vi "Picture_Init_Size.vi"(8 "Input Cluster":T6) -> (0 "Output Cluster":T6, 3 "Boolean":bool)   [LabVIEW 2009]
uses:
  atmcd32d.llb/AcquisitionMode_mode typedef.ctl
  atmcd32d.llb/ReadMode_mode typedef.ctl
  atmcd32d.llb/TriggerMode_mode typedef.ctl
  atmcd32d.llb/Shutter_type typedef.ctl
  atmcd32d.llb/Shutter_mode typedef.ctl
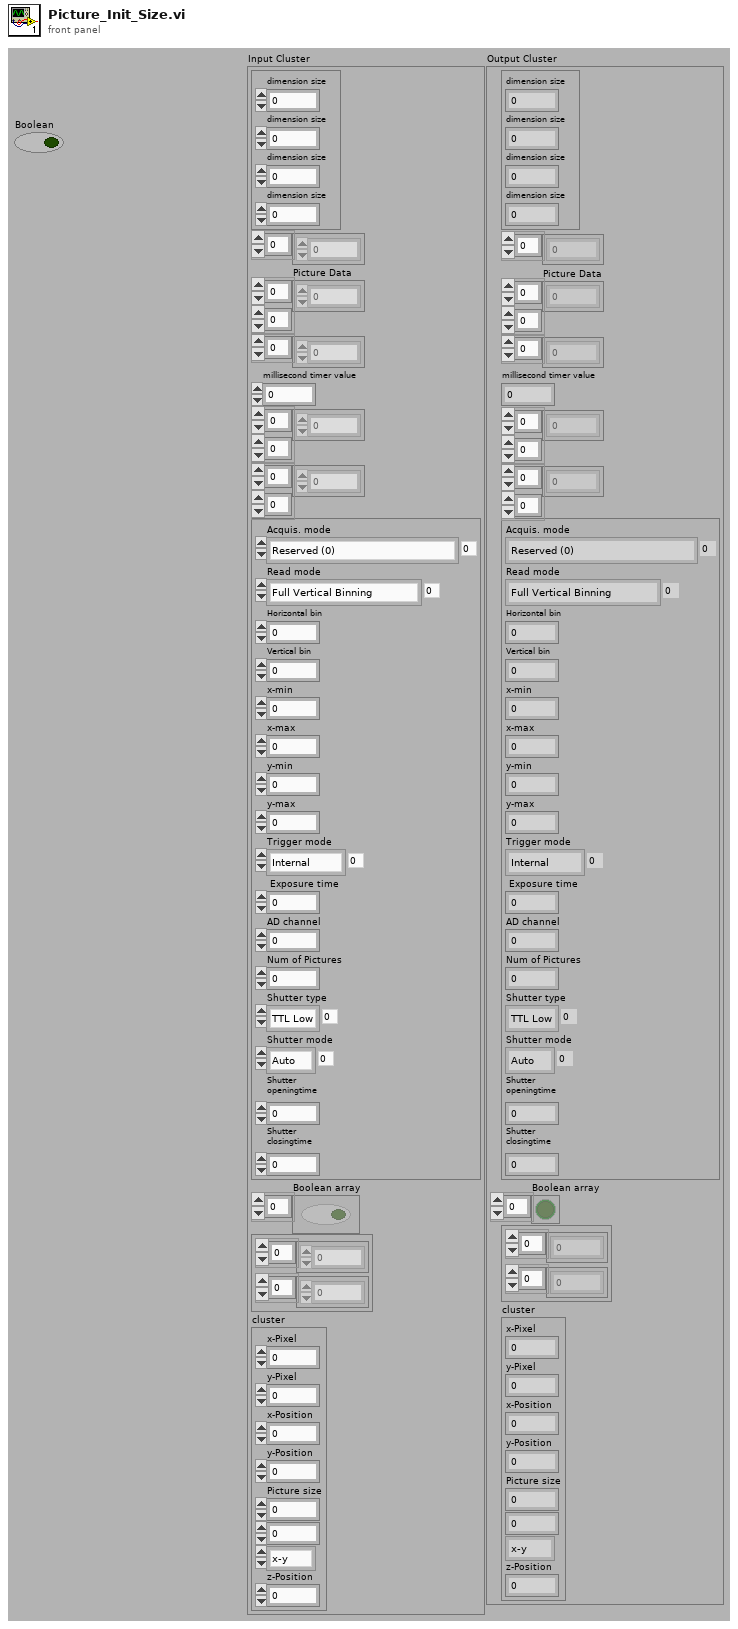
[diagram p1: front panel]
types:
  T1 = typedef "AcquisitionMode_mode typedef.ctl" = enum16{"Reserved (0)", "Single Scan", "Accumulate", "Kinetics", "Fast Kinetics", "Run Till Abort", "Reserved (6)", "Reserved (7)", "Reserved (8)", "Time Delayed Integration"}
  T2 = typedef "ReadMode_mode typedef.ctl" = enum16{"Full Vertical Binning", "Multi-Track", "Random-Track", "Single-Track", "Image"}
  T3 = typedef "TriggerMode_mode typedef.ctl" = enum16{"Internal", "External", "N/A (2)", "N/A (3)", "N/A (4)", "N/A (5)", "External Start"}
  T4 = typedef "Shutter_type typedef.ctl" = enum16{"TTL Low", "TTL High"}
  T5 = typedef "Shutter_mode typedef.ctl" = enum16{"Auto", "Open", "Close"}
  T6 = cluster{cluster{"dimension size":i32, "dimension size":i32, "dimension size":i32, "dimension size":i32}, i32[], "Picture Data":dbl[][], u32[], "millisecond timer value":u32, dbl[][], i32[][], cluster{"Acquis. mode":T1, "Read mode":T2, "Horizontal bin":i32, "Vertical bin":i32, "x-min":i32, "x-max":i32, "y-min":i32, "y-max":i32, "Trigger mode":T3, " Exposure time":sgl, "AD channel":i32, "Num of Pictures":i32, "Shutter type":T4, "Shutter mode":T5, "Shutter\nopeningtime":i32, "Shutter\nclosingtime":i32}, "Boolean array":bool[], cluster{dbl[], dbl[]}, "cluster":cluster{"x-Pixel":u16, "y-Pixel":u16, "x-Position":dbl, "y-Position":dbl, "Picture size":dbl, dbl, enum32{"x-y", "x-z", "y-z"}, "z-Position":dbl}}
  T7 = cluster{"x-Pixel":u16, "y-Pixel":u16, "x-Position":dbl, "y-Position":dbl, "Picture size":dbl, dbl, enum32{"x-y", "x-z", "y-z"}, "z-Position":dbl}
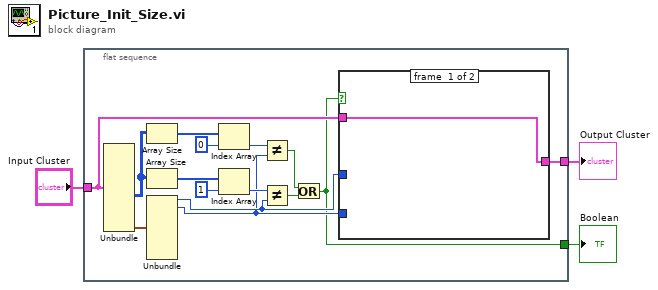
[diagram p0: block diagram]
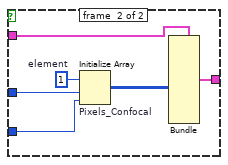
[diagram p2: hidden frame]
diagram:
  n1 = flat-sequence {
    tunnel: "Input Cluster" -> [w7]
    tunnel: [w6] -> w2
    tunnel: [w5] -> w3
    frame #0 {
      n2 = Unbundle(w7) -> (w13:i32[][], "cluster"=w4:T7)  [unwired: 9 out]
      n3 = Array Size(array=w13) -> (size(s)=w15:i32[])
      n4 = Array Size(array=w13) -> (size(s)=w18:i32[])
      n5 = Unbundle(w4) -> ("x-Pixel"=w9:u16, "y-Pixel"=w8:u16)  [unwired: 6 out]
      n6 = Index Array(array=w15, index=0) -> (element=w12:i32)
      n7 = Index Array(array=w18, index=1) -> (element=w16:i32)
      n8 = Not Equal?(x=w12, y=w8) -> (x != y?=w11:bool)
      n9 = Not Equal?(x=w16, y=w9) -> (x != y?=w10:bool)
      n10 = Or(x=w11, y=w10) -> (x .or. y?=w5:bool)
      n11 = case shown="True" w5 {
        tunnel: w9 -> [_ w24]
        tunnel: w8 -> [_ w23]
        tunnel: w7 -> [w19 w22]
        tunnel: [w19 w20] -> w6
        frame #0 {
        }
        frame #1 {
          w25 = 1  # element
          n12 = Initialize Array "Pixels_Confocal"(w25, w24, w23) -> (w21:i32[][])
          n13 = Bundle(cluster=w22, w21) -> (w20:T6)  [unwired: 10 out]
        }
      }
    }
  }
  "Boolean" <- w3
  "Output Cluster" <- w2
